vi "read from json.vi"() -> ()   [LabVIEW 2020]
panel:
  out "Array":T1(array[cluster])
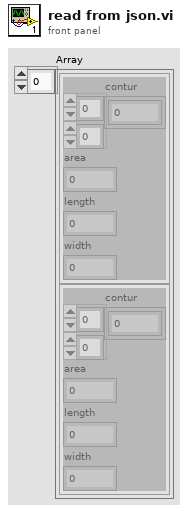
[diagram p1: front panel]
types:
  T1 = cluster{"contur":i32[][], "area":i32, "length":i32, "width":i32}[]
  T2 = cluster{"contur":i32[][], "area":i32, "length":i32, "width":i32}
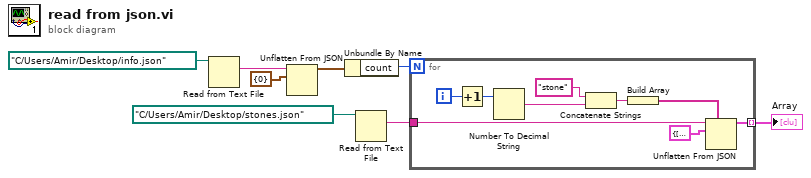
[diagram p0: block diagram]
diagram:
  n1 = Read from Text File(file (use dialog)=path "C:/Users/Amir/Desktop/info.json") -> (text=w6:string)  [unwired: 3 in, 3 out]
  n2 = Unflatten From JSON(JSON string=w6, type and defaults=cluster{"count":i32} {"count"=0}) -> (value=w4:cluster{"count":i32})  [unwired: 5 in, 1 out]
  n3 = Unbundle By Name(w4) -> ("count"=w3:i32)
  n4 = Read from Text File(file (use dialog)=path "C:/Users/Amir/Desktop/stones.json") -> (text=w2:string)  [unwired: 3 in, 3 out]
  n5 = for {
    N: w3 -> [_]
    tunnel: w2 -> [w13]
    tunnel: [w9] -> w1 mode=indexing
    i -> [w16]
    n6 = Increment(x=w16) -> (x+1=w15:i32)
    n7 = Number To Decimal String(number=w15) -> (decimal integer string=w14:string)  [unwired: 1 in]
    n8 = Concatenate Strings("stone" ("string"), w14) -> (w11:string)
    n9 = Build Array(w11) -> (w10:string[])
    n10 = Unflatten From JSON(path=w10, JSON string=w13, type and defaults=T2 {"contur"=[], "area"=0, "length"=0, "width"=0}) -> (value=w9:T2)  [unwired: 4 in, 1 out]
  }
  "Array" <- w1
